vi "CRYAPI Model DOCKING.vi"(8 "sData":string, 9 "nDWinID":i32, 10 "nSWinID":i32, 11 "sAction":string) -> (0 "nData_Out":i32, 1 "sData_Out":string, 2 "tFrame_Out":T2)   [LabVIEW 2013]
uses:
  <vilib>/Utility/miscctls.llb/LVRectTypeDef.ctl
  CRYMain Sub Window Global.vi
panel:
  in  "nDocumentID":i32
  out "bResult":bool=TRUE
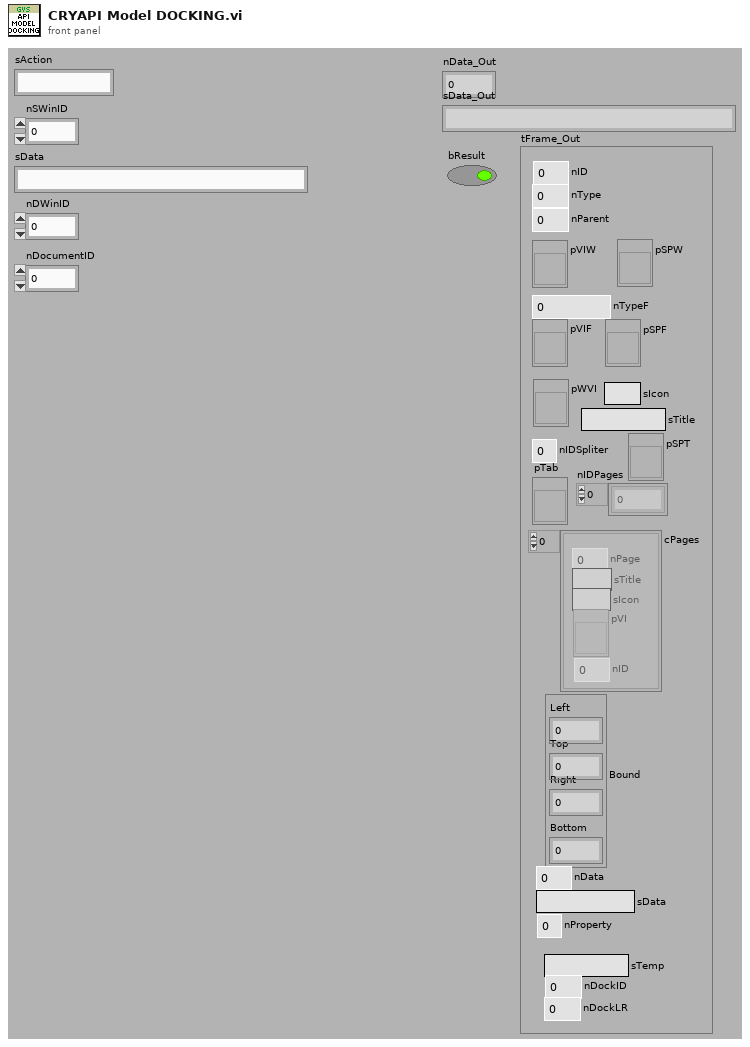
[diagram p1: front panel]
types:
  T1 = typedef "LVRectTypeDef.ctl" = cluster{"Left":i16, "Top":i16, "Right":i16, "Bottom":i16}
  T2 = cluster{"nType":i32, "nParent":i32, "pVIW":refnum<vi>, "pSPW":refnum<vi>, "nTypeF":i32, "pVIF":refnum<vi>, "pSPF":refnum<vi>, "nIDSpliter":i32, "nProperty":i32, "Bound":T1, "nID":i32, "nData":i32, "sData":string, "pWVI":refnum<vi>, "sTitle":string, "cPages":cluster{"nPage":i32, "sTitle":string, "sIcon":string, "pVI":refnum<vi>, "nID":i32}[], "pTab":refnum<vi>, "nIDPages":i32[], "pSPT":refnum<vi>, "sTemp":string, "nDockID":i32, "nDockLR":i32, "sIcon":string}
  T3 = enum32{"Invalid", "Standard", "Closed", "Hidden", "Minimized", "Maximized"}
  T4 = cluster{"nType":i32, "nTypeP":i32, "pVI":refnum<vi>, "pSpliter":refnum<vi>, "pSPL":refnum<vi>, "pVIL":refnum<vi>, "pSPR":refnum<vi>, "pVIR":refnum<vi>, "nIDTL":i32, "nIDL":i32, "nIDTR":i32, "nIDR":i32, "nID":i32, "nIDParent":i32, "nData":i32, "sData":string}
  T5 = cluster{"CLOSE_HIDE":i32, "CLOSE_CLOSE":i32, "DOCK_ENABLE":i32, "DOCK_DISABLE":i32, "FOCUS_SHOW":i32, "FOCUS_HIDE":i32}
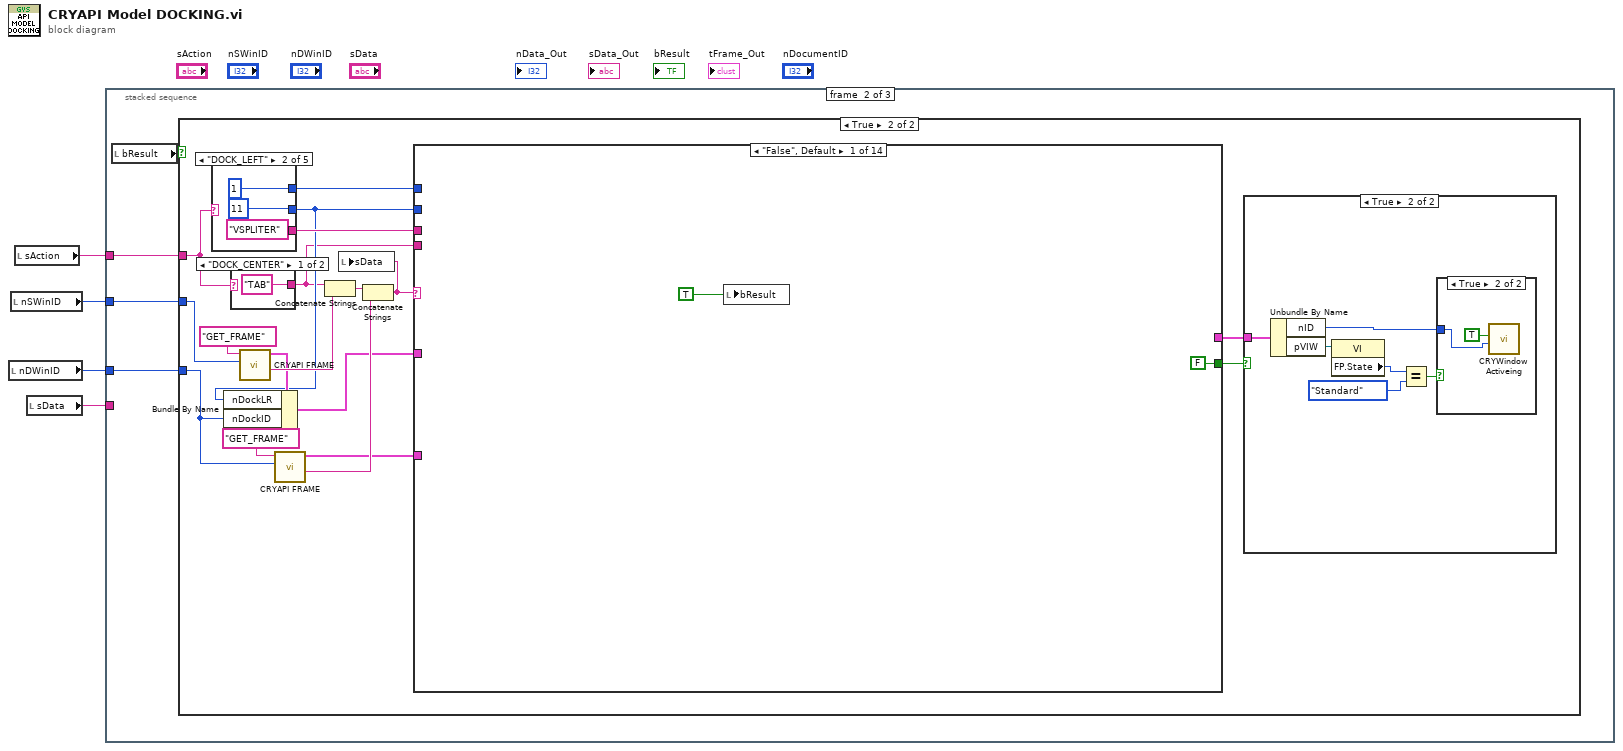
[diagram p0: block diagram]
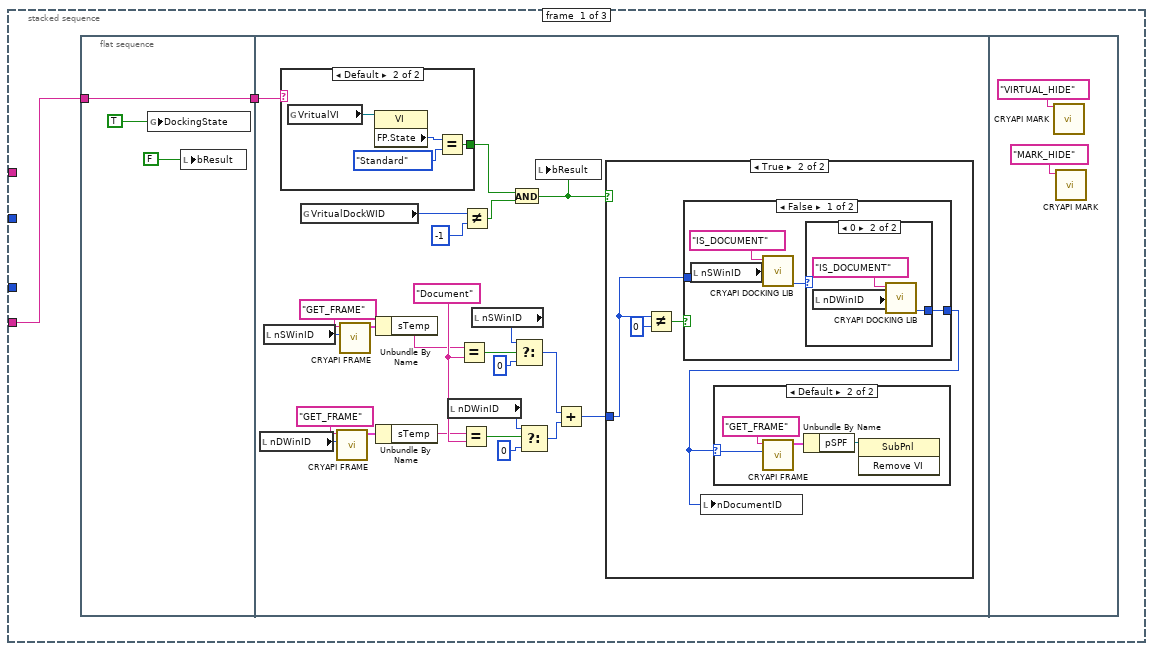
[diagram p2: hidden frame]
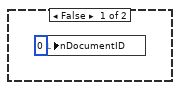
[diagram p3: hidden frame]
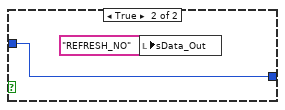
[diagram p6: hidden frame]
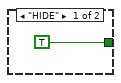
[diagram p7: hidden frame]
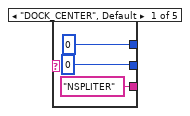
[diagram p11: hidden frame]
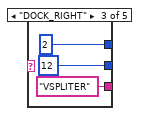
[diagram p12: hidden frame]
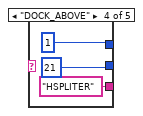
[diagram p13: hidden frame]
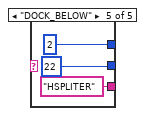
[diagram p14: hidden frame]
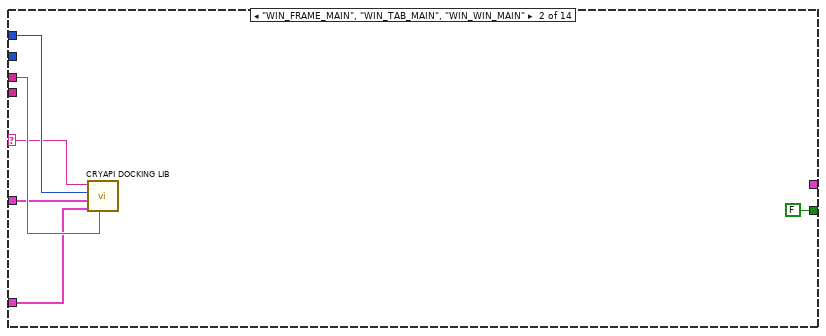
[diagram p15: hidden frame]
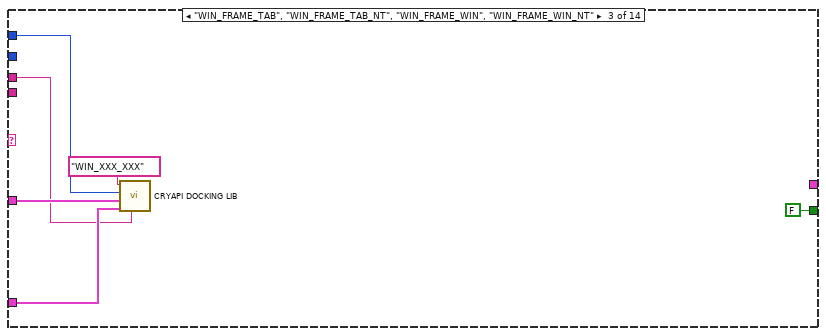
[diagram p16: hidden frame]
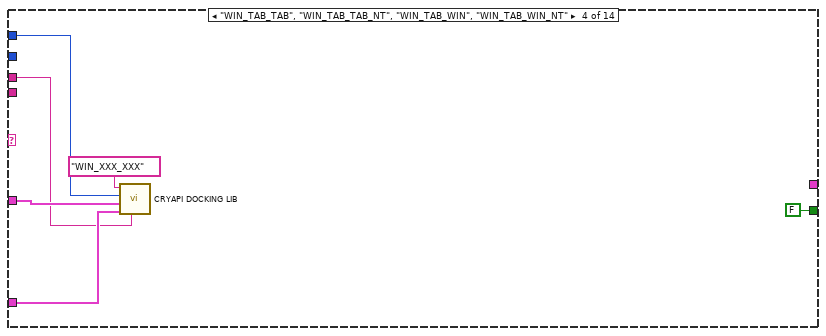
[diagram p17: hidden frame]
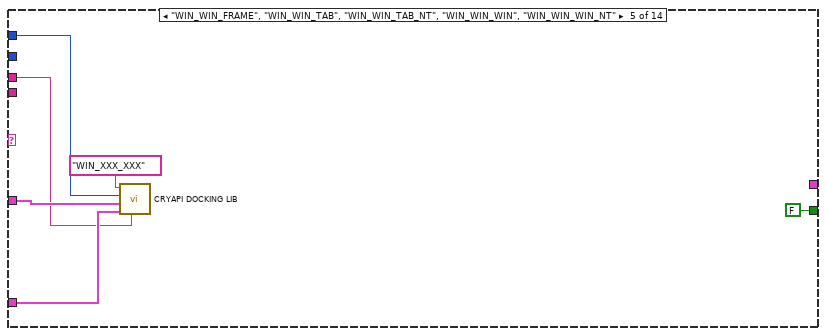
[diagram p18: hidden frame]
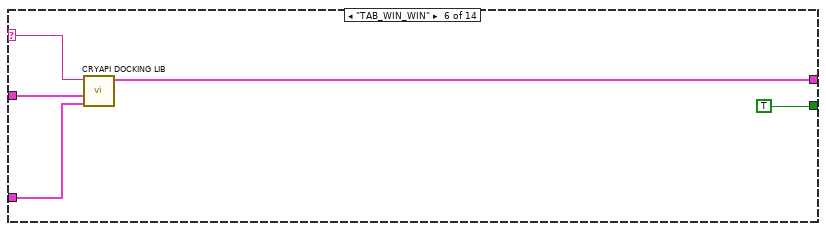
[diagram p19: hidden frame]
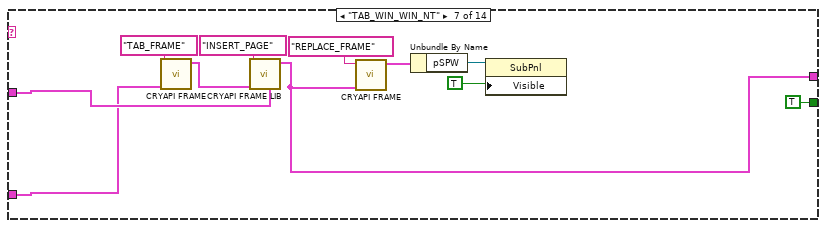
[diagram p20: hidden frame]
diagram:
  n1 = local read "nDWinID"() -> (w2:i32)
  n2 = local read "nSWinID"() -> (w3:i32)
  n3 = local read "sAction"() -> (w4:string)
  n4 = local read "sData"() -> (w1:string)
  n5 = stacked-sequence {
    tunnel: w3 -> [_ w63 w262]
    tunnel: w2 -> [_ w62 w264]
    tunnel: w4 -> [_ w61 w263]
    tunnel: w1 -> [w6 _ _]
    frame #0 {
      n6 = flat-sequence {
        tunnel: w6 -> [w7]
        tunnel: [w7] -> w5
        tunnel: w5 -> [w29]
        frame #0 {
          n7 = global write "CRYMain Sub Window Global.vi" "DockingState"(TRUE ("Docking_State")) -> ()
          n8 = local write "bResult"(FALSE ("bResult")) -> ()
        }
        frame #1 {
          w28 = "Document" ("Window Type")
          n9 = local read "nDWinID"() -> (w14:i32)
          n10 = local read "nSWinID"() -> (w13:i32)
          n11 = case shown="Default" w29 {
            tunnel: [TRUE w54] -> w30
            frame "HIDE" {
            }
            frame Default {
              n12 = global read "CRYMain Sub Window Global.vi" "VritualVI"() -> (w57:refnum<vi>)
              n13 = property class="VI"(reference=w57) -> ("FP.State"=w56:T3)  [unwired: 1 in, 2 out]
              n14 = Equal?(x=w56, y=T3."Standard" ("Front Panel Window:State")) -> (x = y?=w54:bool)
            }
          }
          n15 = global read "CRYMain Sub Window Global.vi" "VritualDockWID"() -> (w32:i32)
          n16 = call "CRYAPI FRAME.vi"("nData"=w14, "sAction"="GET_FRAME") -> ("tFrame_Out"=w17:T2)  [unwired: 4 in, 5 out]
          n17 = call "CRYAPI FRAME.vi"("nData"=w13, "sAction"="GET_FRAME") -> ("tFrame_Out"=w16:T2)  [unwired: 4 in, 5 out]
          n18 = Unbundle By Name(w16) -> ("sTemp"=w18:string)
          n19 = Unbundle By Name(w17) -> ("sTemp"=w19:string)
          n20 = local read "nDWinID"() -> (w23:i32)
          n21 = Equal?(x=w18, y=w28) -> (x = y?=w20:bool)
          n22 = Equal?(x=w19, y=w28) -> (x = y?=w24:bool)
          n23 = Not Equal?(x=w32, y=-1) -> (x != y?=w33:bool)
          n24 = local read "nSWinID"() -> (w11:i32)
          n25 = And(x=w30, y=w33) -> (x .and. y?=w10:bool)
          n26 = Select(t=w11, s=w20, f=0) -> (s? t:f=w25:i32)
          n27 = Select(t=w23, s=w24, f=0) -> (s? t:f=w26:i32)
          n28 = local write "bResult"(w10) -> ()
          n29 = Add(x=w25, y=w26) -> (x+y=w27:i32)
          n30 = case shown="True" w10 {
            tunnel: w27 -> [_ w37]
            frame False {
              n31 = local write "nDocumentID"(0 ("nDocumentID")) -> ()
            }
            frame True {
              n32 = Not Equal?(x=w37, y=0) -> (x != y?=w35:bool)
              n33 = case shown="False" w35 {
                tunnel: w37 -> [_ w52]
                tunnel: [w43 w52] -> w38
                frame False {
                  n34 = local read "nSWinID"() -> (w45:i32)
                  n35 = call "CRYAPI DOCKING LIB.vi"("nData"=w45, "sAction"="IS_DOCUMENT") -> ("nData_Out"=w44:i32)  [unwired: 3 in, 6 out]
                  n36 = case shown="0" w44 {
                    selector: w44 -> [w47 _]
                    tunnel: [w47 w48] -> w43
                    frame Default {
                    }
                    frame 0 {
                      n37 = local read "nDWinID"() -> (w50:i32)
                      n38 = call "CRYAPI DOCKING LIB.vi"("nData"=w50, "sAction"="IS_DOCUMENT") -> ("nData_Out"=w48:i32)  [unwired: 3 in, 6 out]
                    }
                  }
                }
                frame True {
                  n39 = local write "sData_Out"("REFRESH_NO" ("sData_Out")) -> ()
                }
              }
              n40 = local write "nDocumentID"(w38) -> ()
              n41 = case shown="Default" w38 {
                selector: w38 -> [_ w39]
                frame 0 {
                }
                frame Default {
                  n42 = call "CRYAPI FRAME.vi"("nData"=w39, "sAction"="GET_FRAME") -> ("tFrame_Out"=w41:T2)  [unwired: 4 in, 5 out]
                  n43 = Unbundle By Name(w41) -> ("pSPF"=w42:refnum<vi>)
                  n44 = invoke class="SubPnl" method="Remove VI"(reference=w42) -> ()  [unwired: 2 in, 3 out]
                }
              }
            }
          }
        }
        frame #2 {
          n45 = call "CRYAPI MARK.vi"("sAction"="VIRTUAL_HIDE") -> ()  [unwired: 3 in, 7 out]
          n46 = call "CRYAPI MARK.vi"("sAction"="MARK_HIDE") -> ()  [unwired: 3 in, 7 out]
        }
      }
    }
    frame #1 {
      n47 = local read "bResult"() -> (w60:bool)
      n48 = case shown="True" w60 {
        tunnel: w63 -> [_ w74]
        tunnel: w62 -> [_ w68]
        tunnel: w61 -> [_ w72]
        frame False {
        }
        frame True {
          n49 = case shown="\"DOCK_LEFT\"" w72 {
            tunnel: [0 11 12 21 22] -> w67
            tunnel: ["NSPLITER" ("sAction") "VSPLITER" ("sAction") "VSPLITER" ("sAction") "HSPLITER" ("sAction") "HSPLITER" ("sAction")] -> w73
            tunnel: [0 1 2 1 2] -> w71
            frame "DOCK_CENTER", Default {
            }
            frame "DOCK_LEFT" {
            }
            frame "DOCK_RIGHT" {
            }
            frame "DOCK_ABOVE" {
            }
            frame "DOCK_BELOW" {
            }
          }
          n50 = case shown="\"DOCK_CENTER\"" w72 {
            tunnel: ["TAB" ("sAction") "WIN" ("sData")] -> w66
            frame "DOCK_CENTER" {
            }
            frame Default {
            }
          }
          n51 = call "CRYAPI FRAME.vi"("nData"=w74, "sAction"="GET_FRAME") -> ("sData_Out"=w79:string, "tFrame_Out"=w70:T2)  [unwired: 4 in, 4 out]
          n52 = Bundle By Name(cluster=w70, "nDockLR"=w67, "nDockID"=w68) -> (w69:T2)
          n53 = call "CRYAPI FRAME.vi"("nData"=w68, "sAction"="GET_FRAME") -> ("sData_Out"=w78:string, "tFrame_Out"=w76:T2)  [unwired: 4 in, 4 out]
          n54 = Concatenate Strings(w66, w79) -> (w77:string)
          n55 = Concatenate Strings(w77, w78) -> (w75:string)
          n56 = local write "sData"(w75) -> ()
          n57 = case shown="\"False\", Default" w75 {
            selector: w75 -> [_ w108 _ _ _ w134 _ _ w170 _ w187 w191 _ _]
            tunnel: w67 -> [_ _ _ _ _ _ _ _ _ _ _ _ _ _]
            tunnel: w69 -> [_ w109 w117 w123 w129 w135 w142 w154 w164 w179 w188 w192 w197 w240]
            tunnel: w76 -> [_ w111 w118 w124 w130 w133 w141 w152 w165 w183 w185 w189 w199 w245]
            tunnel: w73 -> [_ w112 w115 w121 w127 _ _ _ _ _ _ _ _ _]
            tunnel: w71 -> [_ w110 w116 w122 w128 _ _ _ _ _ _ _ _ _]
            tunnel: w66 -> [_ _ _ _ _ _ _ _ _ _ _ _ _ _]
            tunnel: [_ _ _ _ _ w132 w137 w148 w163 w176 w185 w189 w194 w237] -> w64
            tunnel: [FALSE FALSE FALSE FALSE FALSE TRUE TRUE w147 w162 TRUE TRUE TRUE w193 w236] -> w65
            frame "False", Default {
              n58 = local write "bResult"(TRUE ("bResult")) -> ()
            }
            frame "WIN_FRAME_MAIN", "WIN_TAB_MAIN", "WIN_WIN_MAIN" {
              n59 = call "CRYAPI DOCKING LIB.vi"("sData"=w112, "tDFrame"=w111, "tSFrame"=w109, "nData"=w110, "sAction"=w108) -> ()  [unwired: 7 out]
            }
            frame "WIN_FRAME_TAB", "WIN_FRAME_TAB_NT", "WIN_FRAME_WIN", "WIN_FRAME_WIN_NT" {
              n60 = call "CRYAPI DOCKING LIB.vi"("sData"=w115, "tDFrame"=w118, "tSFrame"=w117, "nData"=w116, "sAction"="WIN_XXX_XXX") -> ()  [unwired: 7 out]
            }
            frame "WIN_TAB_TAB", "WIN_TAB_TAB_NT", "WIN_TAB_WIN", "WIN_TAB_WIN_NT" {
              n61 = call "CRYAPI DOCKING LIB.vi"("sData"=w121, "tDFrame"=w124, "tSFrame"=w123, "nData"=w122, "sAction"="WIN_XXX_XXX") -> ()  [unwired: 7 out]
            }
            frame "WIN_WIN_FRAME", "WIN_WIN_TAB", "WIN_WIN_TAB_NT", "WIN_WIN_WIN", "WIN_WIN_WIN_NT" {
              n62 = call "CRYAPI DOCKING LIB.vi"("sData"=w127, "tDFrame"=w130, "tSFrame"=w129, "nData"=w128, "sAction"="WIN_XXX_XXX") -> ()  [unwired: 7 out]
            }
            frame "TAB_WIN_WIN" {
              n63 = call "CRYAPI DOCKING LIB.vi"("tDFrame"=w133, "tSFrame"=w135, "sAction"=w134) -> ("tFrame_Out"=w132:T2)  [unwired: 2 in, 6 out]
            }
            frame "TAB_WIN_WIN_NT" {
              n64 = call "CRYAPI FRAME.vi"("tFrame"=w141, "sAction"="TAB_FRAME") -> ("tFrame_Out"=w143:T2)  [unwired: 4 in, 5 out]
              n65 = call "CRYAPI FRAME LIB.vi"("tFrame_In"=w142, "tFrame"=w143, "sAction"="INSERT_PAGE") -> ("tFrame_Out"=w137:T2)  [unwired: 3 in, 5 out]
              n66 = call "CRYAPI FRAME.vi"("tFrame"=w137, "sAction"="REPLACE_FRAME") -> ("tFrame_Out"=w140:T2)  [unwired: 4 in, 5 out]
              n67 = Unbundle By Name(w140) -> ("pSPW"=w138:refnum<vi>)
              n68 = property class="SubPnl"(reference=w138, "Visible"=TRUE) -> ()  [unwired: 1 in, 2 out]
            }
            frame "TAB_WIN_TAB", "TAB_WIN_TAB_NT" {
              n69 = call "CRYAPI TAB LIB.vi"("tFrame"=w152, "sAction"="GET_FREE_PAGES") -> ("nData_Out"=w150:i32)  [unwired: 2 in, 7 out]
              n70 = Greater?(x=w150, y=0) -> (0:w151:bool)
              n71 = case shown="True" w151 {
                tunnel: w154 -> [_ w161]
                tunnel: w152 -> [_ w158]
                tunnel: [_ w157] -> w148
                tunnel: [FALSE TRUE] -> w147
                frame False {
                }
                frame True {
                  n72 = call "CRYAPI FRAME LIB.vi"("tFrame_In"=w161, "tFrame"=w158, "sAction"="INSERT_PAGE") -> ("tFrame_Out"=w157:T2)  [unwired: 3 in, 5 out]
                  n73 = call "CRYAPI FRAME.vi"("tFrame"=w157, "sAction"="REPLACE_FRAME") -> ()  [unwired: 4 in, 6 out]
                }
              }
            }
            frame "TAB_TAB_WIN" {
              n74 = call "CRYAPI TAB LIB.vi"("tFrame"=w164, "sAction"="GET_FREE_PAGES") -> ("nData_Out"=w168:i32)  [unwired: 2 in, 7 out]
              n75 = Greater?(x=w168, y=0) -> (0:w166:bool)
              n76 = case shown="True" w166 {
                tunnel: w164 -> [_ w175]
                tunnel: w170 -> [_ w174]
                tunnel: w165 -> [_ w172]
                tunnel: [_ w172] -> w163
                tunnel: [FALSE TRUE] -> w162
                frame False {
                }
                frame True {
                  n77 = call "CRYAPI DOCKING LIB.vi"("tDFrame"=w172, "tSFrame"=w175, "sAction"=w174) -> ()  [unwired: 2 in, 7 out]
                }
              }
            }
            frame "TAB_TAB_WIN_NT" {
              n78 = call "CRYAPI FRAME.vi"("tFrame"=w183, "sAction"="TAB_FRAME") -> ("tFrame_Out"=w176:T2)  [unwired: 4 in, 5 out]
              n79 = call "CRYAPI DOCKING LIB.vi"("tDFrame"=w176, "tSFrame"=w179, "sAction"="TAB_TAB_TAB") -> ("tFrame_Out"=w178:T2)  [unwired: 2 in, 6 out]
              n80 = Unbundle By Name(w178) -> ("pSPW"=w180:refnum<vi>)
              n81 = property class="SubPnl"(reference=w180, "Visible"=TRUE) -> ()  [unwired: 1 in, 2 out]
            }
            frame "TAB_TAB_TAB", "TAB_TAB_TAB_NT" {
              n82 = call "CRYAPI DOCKING LIB.vi"("tDFrame"=w185, "tSFrame"=w188, "sAction"=w187) -> ()  [unwired: 2 in, 7 out]
            }
            frame "TAB_FRAME_TAB", "TAB_FRAME_TAB_NT" {
              n83 = call "CRYAPI DOCKING LIB.vi"("tDFrame"=w189, "tSFrame"=w192, "sAction"=w191) -> ()  [unwired: 2 in, 7 out]
            }
            frame "TAB_FRAME_WIN" {
              n84 = call "CRYAPI REMOVE.vi"("tFrame"=w197, "sAction"="GET_LIST_ID") -> ("List_ID_Out"=w201:i32[])  [unwired: 3 in, 6 out]
              n85 = call "CRYAPI REMOVE.vi"("List_ID"=w201, "sAction"="GET_LIST_IDWIN") -> ("nData_Out"=w195:i32)  [unwired: 3 in, 6 out]
              n86 = Increment(x=w195) -> (x+1=w196:i32)
              n87 = call "CRYAPI TAB LIB.vi"("nData"=w196, "sAction"="CHECK_MAX_PAGES") -> ("nData_Out"=w198:i32)  [unwired: 2 in, 7 out]
              n88 = case shown="1" w198 {
                tunnel: w197 -> [_ w211]
                tunnel: w199 -> [_ w207]
                tunnel: [_ w206] -> w194
                tunnel: [FALSE TRUE] -> w193
                frame 0, Default {
                }
                frame 1 {
                  n89 = Unbundle By Name(w207) -> ("nParent"=w217:i32)
                  n90 = call "CRYAPI FRAME.vi"("sData"="TAB_YTITLE", "sAction"="NEW_FRAME") -> ("tFrame_Out"=w221:T2)  [unwired: 4 in, 5 out]
                  n91 = call "CRYAPI FRAME.vi"("tFrame_In"=w207, "tFrame"=w221, "sAction"="SET_FRAME_CLONE") -> ("tFrame_Out"=w216:T2)  [unwired: 3 in, 5 out]
                  n92 = case shown="Default" w217 {
                    selector: w217 -> [_ w226]
                    tunnel: w216 -> [w225 w228]
                    tunnel: [w225 w227] -> w213
                    tunnel: w207 -> [_ w233]
                    frame 0 {
                    }
                    frame Default {
                      n93 = call "CRYAPI SPLITE.vi"("nData"=w226, "sAction"="GET_SPLITER") -> ("tSpliter_Out"=w232:T4)  [unwired: 4 in, 5 out]
                      n94 = call "CRYAPI SPLITE.vi"("tFrame"=w233, "tSpliter"=w232, "sAction"="GET_FRAME_LR") -> ("nData_Out"=w230:i32, "tSpliter_Out"=w231:T4)  [unwired: 3 in, 4 out]
                      n95 = call "CRYAPI SPLITE LIB.vi"("tFrame"=w228, "tSpliter"=w231, "nData"=w230, "sAction"="EXCHANGE_FRAME_LR") -> ("tFrame_Out"=w227:T2)  [unwired: 2 in, 5 out]
                    }
                  }
                  n96 = call "CRYAPI FRAME LIB.vi"("tFrame_In"=w207, "tFrame"=w213, "sAction"="INSERT_PAGE") -> ("tFrame_Out"=w212:T2)  [unwired: 3 in, 5 out]
                  n97 = call "CRYAPI DOCKING LIB.vi"("tDFrame"=w212, "tSFrame"=w211, "sAction"="TAB_FRAME_TAB") -> ("tFrame_Out"=w208:T2)  [unwired: 2 in, 6 out]
                  n98 = call "CRYAPI FRAME.vi"("tFrame"=w208, "sAction"="ADD_FRAME") -> ("tFrame_Out"=w206:T2)  [unwired: 4 in, 5 out]
                  n99 = Unbundle By Name(w206) -> ("nParent"=w209:i32)
                  n100 = case shown="0" w209 {
                    tunnel: w206 -> [_ w222]
                    frame Default {
                    }
                    frame 0 {
                      n101 = Unbundle By Name(w222) -> ("pVIW"=w223:refnum<vi>)
                      n102 = property class="VI"(reference=w223, "Front Panel.Open"=TRUE ("Front Panel Window:Open")) -> ()  [unwired: 1 in, 2 out]
                    }
                  }
                }
              }
            }
            frame "TAB_FRAME_WIN_NT" {
              n103 = call "CRYAPI REMOVE.vi"("tFrame"=w240, "sAction"="GET_LIST_ID") -> ("List_ID_Out"=w243:i32[])  [unwired: 3 in, 6 out]
              n104 = call "CRYAPI REMOVE.vi"("List_ID"=w243, "sAction"="GET_LIST_IDWIN") -> ("nData_Out"=w238:i32)  [unwired: 3 in, 6 out]
              n105 = call "CRYAPI TAB LIB.vi"("nData"=w238, "sAction"="CHECK_MAX_PAGES") -> ("nData_Out"=w239:i32)  [unwired: 2 in, 7 out]
              n106 = case shown="0, Default" w239 {
                tunnel: w240 -> [_ w254]
                tunnel: w245 -> [_ w253]
                tunnel: [_ w248] -> w237
                tunnel: [FALSE TRUE] -> w236
                frame 0, Default {
                }
                frame 1 {
                  n107 = call "CRYAPI FRAME.vi"("tFrame"=w253, "sAction"="TAB_FRAME") -> ("tFrame_Out"=w256:T2)  [unwired: 4 in, 5 out]
                  n108 = call "CRYAPI DOCKING LIB.vi"("tDFrame"=w256, "tSFrame"=w254, "sAction"="TAB_FRAME_TAB_NT") -> ("tFrame_Out"=w248:T2)  [unwired: 2 in, 6 out]
                  n109 = Unbundle By Name(w248) -> ("pVIF"=w250:refnum<vi>, "pSPW"=w259:refnum<vi>)
                  n110 = invoke class="VI" method="Ctrl Val.Set"(reference=w250, "Control Name"="sMessage", "Value"="REFRESH_PANE" ("sAction")) -> (error out=w249:errorcluster)  [unwired: 2 in, 4 out]
                  n111 = property class="SubPnl"(reference=w259, error in=w249, "Visible"=TRUE) -> ()  [unwired: 2 out]
                }
              }
            }
          }
          n112 = case shown="True" w65 {
            tunnel: w64 -> [_ w82]
            frame False {
            }
            frame True {
              n113 = Unbundle By Name(w82) -> ("nID"=w87:i32, "pVIW"=w83:refnum<vi>)
              n114 = property class="VI"(reference=w83) -> ("FP.State"=w84:T3)  [unwired: 1 in, 2 out]
              n115 = Equal?(x=w84, y=T3."Standard" ("Front Panel Window:State")) -> (x = y?=w86:bool)
              n116 = case shown="True" w86 {
                tunnel: w87 -> [_ w88]
                frame False {
                }
                frame True {
                  n117 = call "CRYWindow Activeing.vi"("nID"=w88, "ActiveTF"=TRUE) -> ()  [unwired: 10 in]
                }
              }
            }
          }
        }
      }
    }
    frame #2 {
      # "Parent is 0:Error 1:MAIN 2:WIN_NT 3:TAB_NT 4:WIN 5:TAB"
      n118 = global write "CRYMain Sub Window Global.vi" "DockingState"(FALSE ("Docking_State")) -> ()
      n119 = flat-sequence {
        tunnel: w264 -> [w279]
        tunnel: w263 -> [w278]
        tunnel: w262 -> [w268]
        frame #0 {
          n120 = call "CRYAPI FRAME.vi"("nData"=w268, "sAction"="FIND_WIN_ID") -> ("nData_Out"=w267:i32, "tFrame_Out"=w270:T2)  [unwired: 4 in, 4 out]
          n121 = call "CRYAPI DOCKING LIB.vi"("sData"=w278, "nData"=w279, "sAction"="CHECK_PARENT") -> ("tFrame_Out"=w277:T2)  [unwired: 2 in, 6 out]
          n122 = global read "CRYMain Sub Window Global.vi" "CounterActive"() -> (w271:i32)
          n123 = local read "nDocumentID"() -> (w266:i32)
          n124 = case shown="Default" w267 {
            tunnel: w270 -> [_ w307]
            frame 0 {
            }
            frame Default {
              n125 = global read "CRYMain Sub Window Global.vi" "tWinType"() -> (w308:T5)
              n126 = Unbundle By Name(w308) -> ("FOCUS_HIDE"=w305:i32)
              n127 = Unbundle By Name(w307) -> ("pVIW"=w303:refnum<vi>, "nProperty"=w306:i32)
              n128 = And(x=w306, y=w305) -> (x .and. y?=w304:i32)
              n129 = case shown="Default" w304 {
                tunnel: w303 -> [_ w310]
                frame 0 {
                }
                frame Default {
                  n130 = call "CRYAPI Get Boolean Reference.vi"("Label Name"="PinTrue", "VI Refnum"=w310) -> ("Boolean Ref"=w311:refnum<vi>)  [unwired: 9 out]
                  n131 = property class="Bool"(reference=w311, "Visible"=FALSE) -> ()  [unwired: 1 in, 2 out]
                }
              }
            }
          }
          n132 = Unbundle By Name(w277) -> ("nTypeF"=w276:i32, "nID"=w275:i32)
          n133 = case shown="Default" w266 {
            selector: w266 -> [_ w283]
            frame 0 {
            }
            frame Default {
              n134 = call "CRYAPI FRAME.vi"("nData"=w283, "sAction"="FIND_WIN_ID") -> ("nData_Out"=w281:i32, "tFrame_Out"=w282:T2)  [unwired: 4 in, 4 out]
              n135 = case shown="Default" w281 {
                tunnel: w282 -> [_ w285]
                frame 0 {
                }
                frame Default {
                  n136 = Unbundle By Name(w285) -> ("nTypeF"=w288:i32)
                  n137 = Equal?(x=w288, y=1) -> (x = y?=w286:bool)
                  n138 = case shown="True" w286 {
                    tunnel: w285 -> [w293 w300]
                    frame False {
                      n139 = Unbundle By Name(w293) -> ("nParent"=w289:i32, "pSPF"=w292:refnum<vi>, "pWVI"=w291:refnum<vi>)
                      n140 = Less Or Equal To 0?(x=w289) -> (x <= 0?=w290:bool)
                      n141 = case shown="True" w290 {
                        tunnel: w292 -> [_ w295]
                        tunnel: w291 -> [_ w294]
                        frame False {
                        }
                        frame True {
                          n142 = invoke class="SubPnl" method="Insert VI"(reference=w295, "VI Ref"=w294) -> ()  [unwired: 2 in, 4 out]
                        }
                      }
                    }
                    frame True {
                      n143 = Unbundle By Name(w300) -> ("pVIF"=w299:refnum<vi>)
                      n144 = call "CRYGet Boolean Reference.vi"("Label Name"="bRefresh", "VI Refnum"=w299) -> ("Exist?"=w296:bool, "Boolean Ref"=w297:refnum<vi>)  [unwired: 8 out]
                      n145 = case shown="True" w296 {
                        tunnel: w297 -> [_ w302]
                        frame False {
                        }
                        frame True {
                          n146 = property class="Bool"(reference=w302, "Val(Sgnl)"=TRUE) -> ()  [unwired: 1 in, 2 out]
                        }
                      }
                    }
                  }
                }
              }
            }
          }
          n147 = case shown="0, Default" w276 {
            tunnel: w277 -> [w317 w329]
            tunnel: [w318 w328] -> w273
            tunnel: w275 -> [w325 _]
            tunnel: [w321 w327] -> w272
            tunnel: w271 -> [w320 w327]
            frame 0, Default {
              n148 = global read "CRYMain Sub Window Global.vi" "MainFrame_nID"() -> (w324:i32)
              n149 = Unbundle By Name(w317) -> ("nID"=w316:i32)
              n150 = call "CRYAPI REMOVE.vi"("tFrame"=w317, "sAction"="GET_LIST_WIN") -> ("List_ID_Out"=w319:i32[])  [unwired: 3 in, 6 out]
              n151 = Equal?(x=w325, y=w324) -> (x = y?=w323:bool)
              n152 = Insert Into Array(array=w319, new element=w316) -> (w318:i32[])  [unwired: 1 in]
              n153 = Select(t=0 ("nData"), s=w323, f=w320) -> (s? t:f=w321:i32)
            }
            frame 1 {
              n154 = Unbundle By Name(w329) -> ("nID"=w330:i32)
              n155 = call "CRYAPI REMOVE.vi"("tFrame"=w329, "sAction"="GET_LIST_PAGES") -> ("List_ID_Out"=w331:i32[])  [unwired: 3 in, 6 out]
              n156 = Insert Into Array(array=w331, new element=w330) -> (w328:i32[])  [unwired: 1 in]
            }
          }
          n157 = Greater Or Equal To 0?(x=w272) -> (x >= 0?=w274:bool)
          n158 = case shown="True" w274 {
            tunnel: w273 -> [_ w314]
            tunnel: w272 -> [_ w313]
            frame False {
            }
            frame True {
              n159 = call "CRYAPI REMOVE.vi"("nData"=w313, "List_ID"=w314, "sAction"="SET_ACTIVENUMBERS") -> ()  [unwired: 2 in, 7 out]
            }
          }
        }
        frame #1 {
          n160 = call "CRYWindow PIC Project State Change.vi"() -> ()  [unwired: 12 in]
          n161 = call "CRYProject Editor PIC Action End.vi"() -> ()  [unwired: 12 in]
        }
      }
    }
  }
